vi "Manual.vi"(7 "vi reference":refnum<vi>, 8 "error in (no error)":errorcluster, 9 "IOList_280":T3, 11 "Manual":T6(tab)) -> (0 "error out":errorcluster, 3 "Out reference":refnum<vi>)   [LabVIEW 2015]
uses:
  Control Button/Exit.ctl
  Control Button/Scanner config.ctl
  Galobal variable_TI.vi
  <vilib>/Instr/_visa.llb/VISA Configure Serial Port (Instr).vi
panel:
  in  "Sensor Setting Data":T1 {"IL Sensor_Max (AI12)" format="%0.02f"; "IL Sensor_Max (AI11)" format="%0.02f"; "IL Sensor_Max (AI10)" format="%0.02f"; "IL Sensor_Max (AI9)" format="%0.02f"; "IL Sensor1_Max AI1" format="%0.02f"; "IL Sensor1_Max AI0" format="%0.02f"; "IL Sensor_Min (AI12" format="%0.02f"; "IL Sensor_Min (AI11)" format="%0.02f"; "IL Sensor_Min(AI10)" format="%0.02f"; "IL Sensor_Min  (AI9)" format="%0.02f"; "IL Sensor1_ Min AI1" format="%0.02f"; "IL Sensor1_Min AI0" format="%0.02f"}
  out "Sensor Data":T2 {"IL Sensor  (AI12" format="%0.02f"; "IL Sensor (AI11)" format="%0.02f"; "IL Sensor  (AI10)" format="%0.02f"; "IL Sensor (AI9)" format="%0.02f"; "IL Sensor1_AI1" format="%0.02f"; "IL Sensor1_AI0" format="%0.02f"}
  out "Array":string[](array[string])
  out "Byte Lenth":i32
  out "error out 2":errorcluster
  out "Manual DO":bool[](array[boolean])
  in  "Stop":T4
  out "NewVal":T5
  in  "Digital Output":T7
  out "LVDT":string
  out "Digital Input":T8
  in  "Home Calling M1":bool
  in  "Stop M1":bool
  in  "SERVO ON CMD M1":bool
  in  "Speed (mm/s) M1":i32=10
  in  "Travel (mm)M1":i32=5
  out "STM1 Done Bit":bool
  out "Error Message":string
  out "Cluster":T9
  out "Error Status":bool
  in  "Scanner config":T10
  out "Read data":string
  out "Boolean":bool
  # "Instruction for Servo motor Operate\n(1)  Switch  ON -OFF  of Fixture Slide servo Brake ON Cmd (P0.19)  \n      from Digital Output tab.\n(2) Switch  ON -OFF  of Fixture Slide Servo Direction Command (P0.20)\n      from Digital Output tab."
  # "Fixture Slide servo"
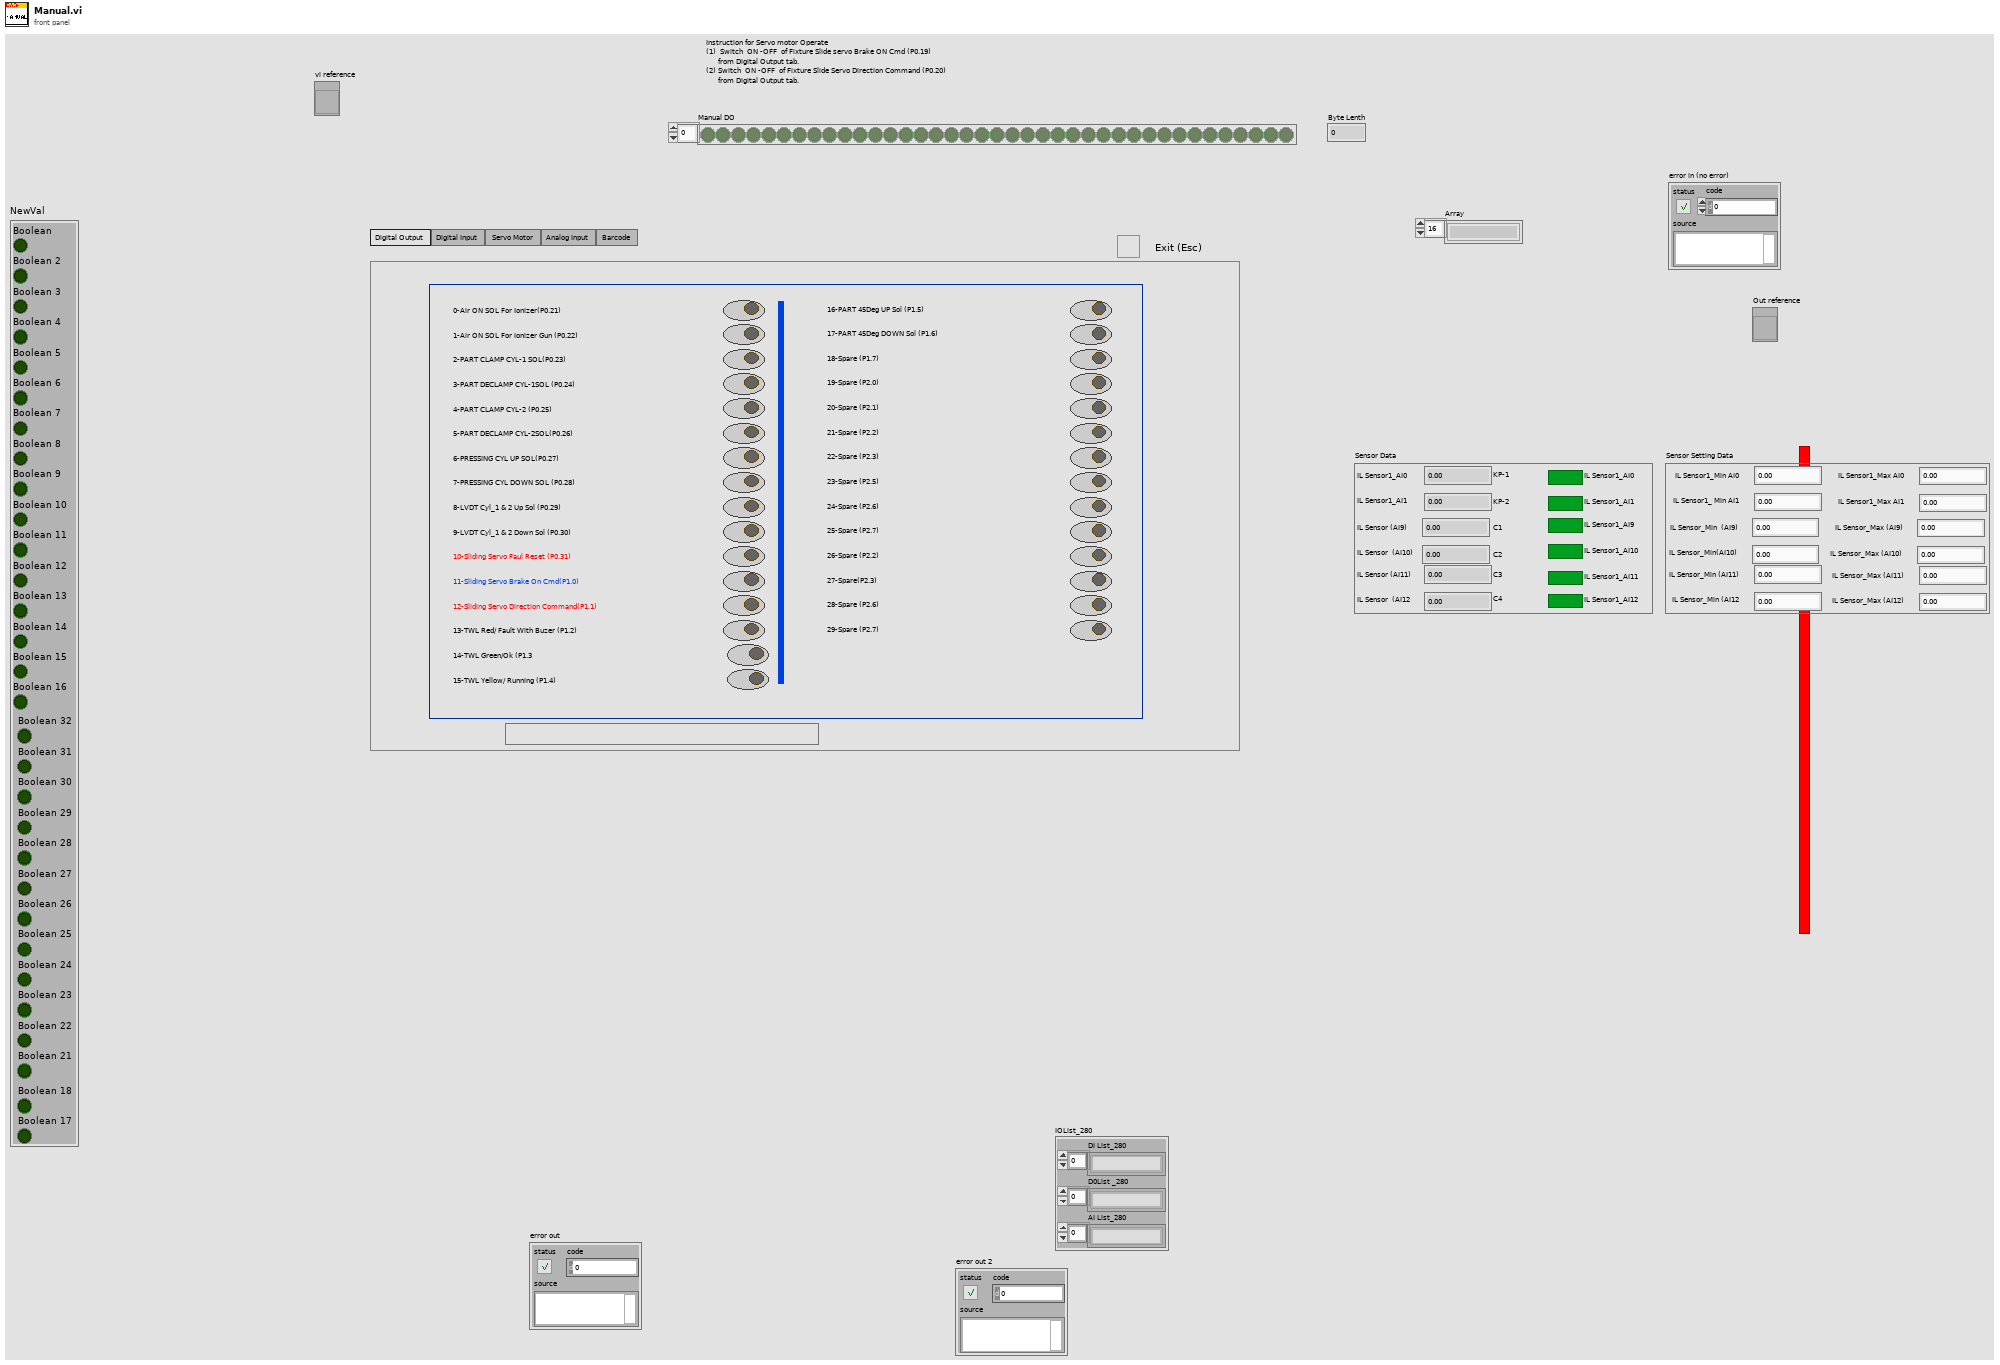
[diagram p1: front panel]
types:
  T1 = cluster{"IL Sensor1_Max AI0":dbl, "IL Sensor1_Min AI0":dbl, "IL Sensor1_Max AI1":dbl, "IL Sensor1_ Min AI1":dbl, "IL Sensor_Max (AI9)":dbl, "IL Sensor_Min  (AI9)":dbl, "IL Sensor_Max (AI10)":dbl, "IL Sensor_Min(AI10)":dbl, "IL Sensor_Max (AI11)":dbl, "IL Sensor_Min (AI11)":dbl, "IL Sensor_Max (AI12)":dbl, "IL Sensor_Min (AI12":dbl}
  T2 = cluster{"IL Sensor1_AI0":dbl, "IL Sensor1_AI1":dbl, "IL Sensor (AI9)":dbl, "IL Sensor  (AI10)":dbl, "IL Sensor (AI11)":dbl, "IL Sensor  (AI12":dbl, "IL Sensor1_AI0":bool, "IL Sensor1_AI1":bool, "IL Sensor1_AI9":bool, "IL Sensor1_AI10":bool, "IL Sensor1_AI11":bool, "IL Sensor1_AI12":bool}
  T3 = cluster{"DI List_280":string[], "D0List _280":string[], "AI List_280":string[]}
  T4 = typedef "Exit.ctl" = bool
  T5 = cluster{"Boolean":bool, "Boolean 2":bool, "Boolean 3":bool, "Boolean 4":bool, "Boolean 5":bool, "Boolean 6":bool, "Boolean 7":bool, "Boolean 8":bool, "Boolean 9":bool, "Boolean 10":bool, "Boolean 11":bool, "Boolean 12":bool, "Boolean 13":bool, "Boolean 14":bool, "Boolean 15":bool, "Boolean 16":bool, "Boolean 17":bool, "Boolean 18":bool, "Boolean 21":bool, "Boolean 22":bool, "Boolean 23":bool, "Boolean 24":bool, "Boolean 25":bool, "Boolean 26":bool, "Boolean 27":bool, "Boolean 28":bool, "Boolean 29":bool, "Boolean 30":bool, "Boolean 31":bool, "Boolean 32":bool}
  T6 = enum32{"Digital Output", "Digital Input", "Servo Motor ", "Analog Input", "Barcode "}
  T7 = cluster{"DO.00":bool, "DO.01":bool, "DO.02":bool, "DO.03":bool, "DO.04":bool, "DO.05":bool, "DO.06":bool, "DO.06":bool, "DO.07":bool, "DO.08":bool, "DO.09":bool, "DO.10":bool, "DO.11":bool, "DO.12":bool, "DO.13":bool, "DO.14":bool, "DO.07 2":bool, "DO.08 2":bool, "DO.09 2":bool, "DO.10 2":bool, "DO.11 2":bool, "DO.12 2":bool, "DO.13 2":bool, "DO.14 2":bool, "DO.00 2":bool, "DO.01 2":bool, "DO.02 2":bool, "DO.03 2":bool, "DO.06 2":bool, "DO.06 3":bool}
  T8 = cluster{"Digital Input":bool, "Digital Input 2":bool, "Digital Input 3":bool, "Digital Input 4":bool, "Digital Input 5":bool, "Digital Input 6":bool, "Digital Input 7":bool, "Digital Input 8":bool, "Digital Input 9":bool, "Digital Input 10":bool, "Digital Input 11":bool, "Digital Input 12":bool, "Digital Input 13":bool, "Digital Input 14":bool, "Digital Input 15":bool, "Digital Input 16":bool, "Digital Input 17":bool, "Digital Input 18":bool, "Digital Input 19":bool, "Digital Input 20":bool, "Digital Input 21":bool, "Digital Input 22":bool, "Digital Input 23":bool, "Digital Input 24":bool, "Digital Input 25":bool, "Digital Input 26":bool, "Digital Input 27":bool, "Digital Input 28":bool, "Digital Input 29":bool, "Digital Input 30":bool, "Digital Input 31":bool, "Digital Input 32":bool, "Digital Input 33":bool, "Digital Input 34":bool, "Digital Input 35":bool, "Digital Input 36":bool, "Digital Input 37":bool, "Digital Input 38":bool, "Digital Input 39":bool, "Digital Input 40":bool, "Digital Input 41":bool, "Digital Input 42":bool, "Digital Input 43":bool, "Digital Input 44":bool}
  T9 = cluster{"Load Cell (AI0)":dbl, "LVDT (AI1)":dbl, "LVDT (AI2)":dbl}
  T10 = typedef "Scanner config.ctl" = bool
  T11 = cluster{" Fixture Brack on":refnum<vi>, " Fixture Direction":refnum<vi>, "Servo Cmd":refnum<vi>, "Servo Home":refnum<vi>}
  T12 = cluster{"VISA resource name":refnum<visa-resource-name>, "baud rate ":u32}
  T13 = cluster{"Emergency_1":bool, "Reset_2":bool, "Home _3":bool, "Air Pressure_4":bool, "Safety Sensor_5":bool, "Safety Sensor_6":bool, "Slide Servo Home RS 26":bool, "LVDT UP RS":bool, "Servo Fault 27":bool, "Pressing UP RS 31":bool, "40 Deg. Down Fixture Rs":bool}
  T14 = cluster{"IL Sensor1_AI0":dbl, "IL Sensor1_AI1":dbl, "IL Sensor (AI6)":dbl, "IL Sensor  (AI7)":dbl, "IL Sensor (AI8)":dbl, "IL Sensor  (AI9)":dbl, "IL Sensor1_AI0":bool, "IL Sensor1_AI1":bool, "IL Sensor1_AI9":bool, "IL Sensor1_AI10":bool, "IL Sensor1_AI11":bool, "IL Sensor1_AI12":bool}
  T15 = cluster{"Digital input[0]":bool, "Digital input[1]":bool, "Digital input[2]":bool, "Digital input[3]":bool, "Digital input[4]":bool, "Digital input[5]":bool, "Digital input[6]":bool, "Digital input[7]":bool, "Digital input[8]":bool, "Digital input[9]":bool, "Digital input[10]":bool, "Digital input[11]":bool, "Digital input[12]":bool, "Digital input[13]":bool, "Digital input[14]":bool, "Digital input[15]":bool, "Digital input[16]":bool, "Digital input[17]":bool, "Digital input[18]":bool, "Digital input[19]":bool, "Digital input[20]":bool, "Digital input[21]":bool, "Digital input[22]":bool, "Digital input[23]":bool, "Digital input[24]":bool, "Digital input[25]":bool, "Digital input[26]":bool, "Digital input[27]":bool, "Digital input[28]":bool, "Digital input[29]":bool, "Digital input[30]":bool, "Digital input[31]":bool, "Digital input[32]":bool, "Digital input[33]":bool, "Digital input[34]":bool, "Digital input[35]":bool, "Digital input[36]":bool, "Digital input[37]":bool, "Digital input[38]":bool, "Digital input[39]":bool, "Digital input[40]":bool, "Digital input[41]":bool, "Digital input[42]":bool, "Digital input[43]":bool}
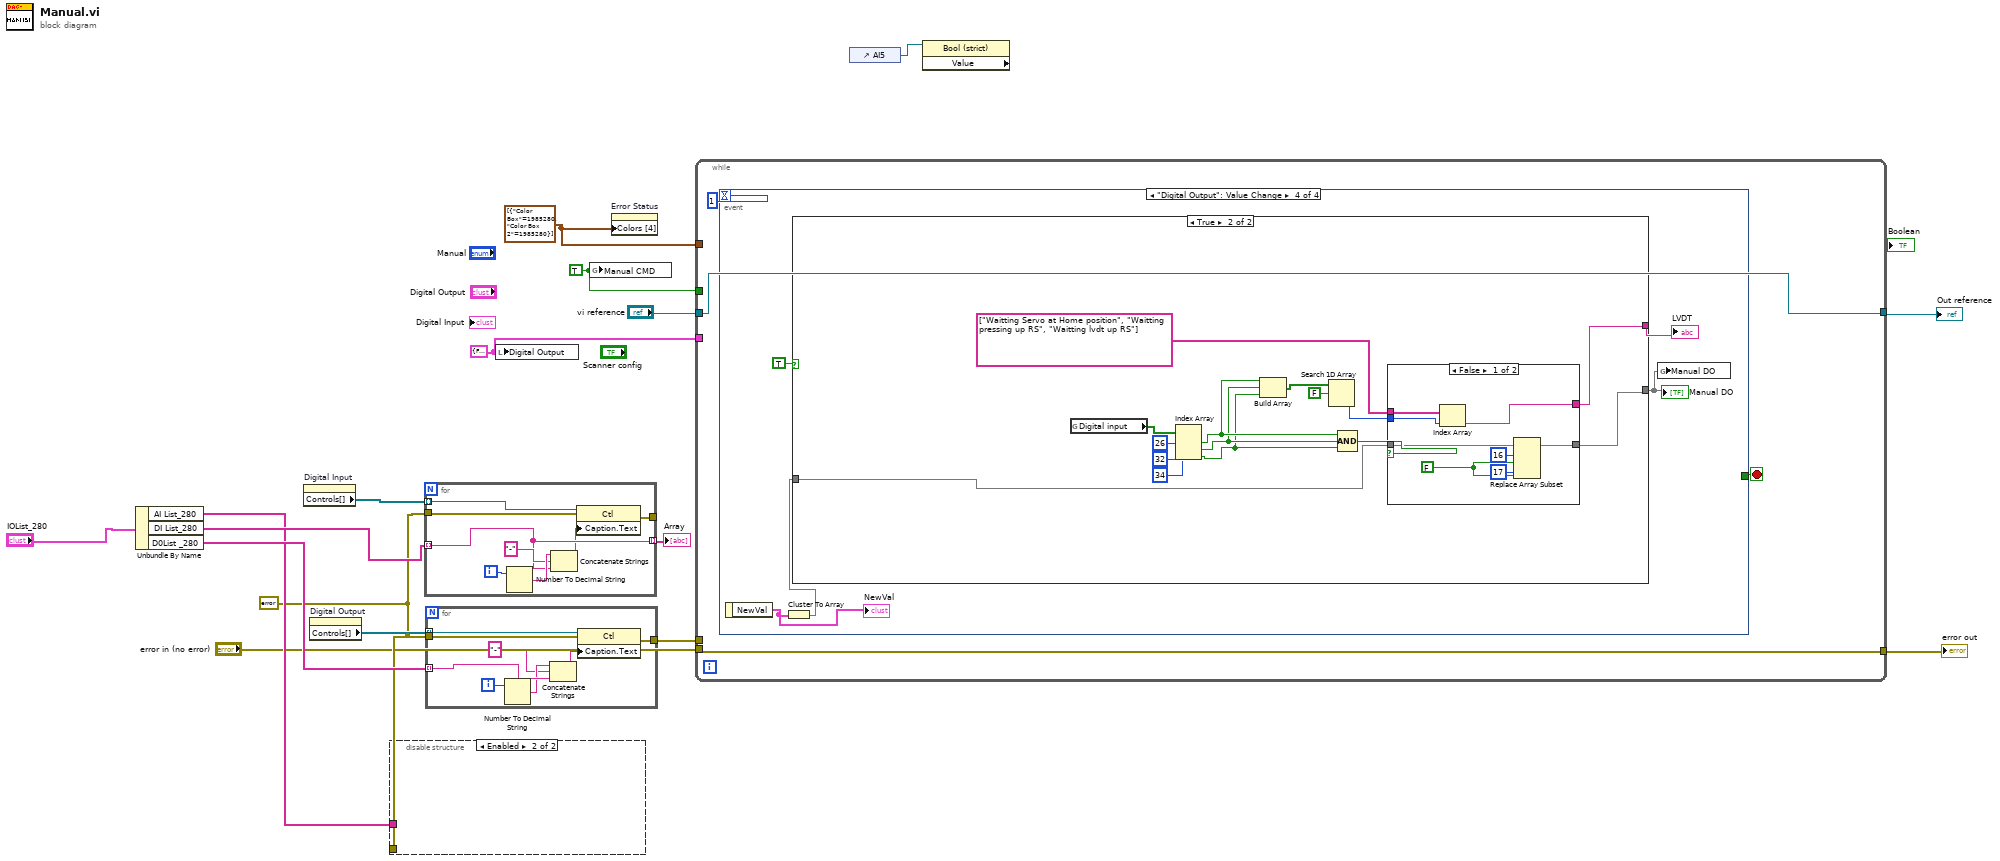
[diagram p0: block diagram]
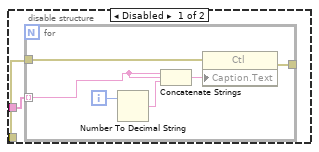
[diagram p2: hidden frame]
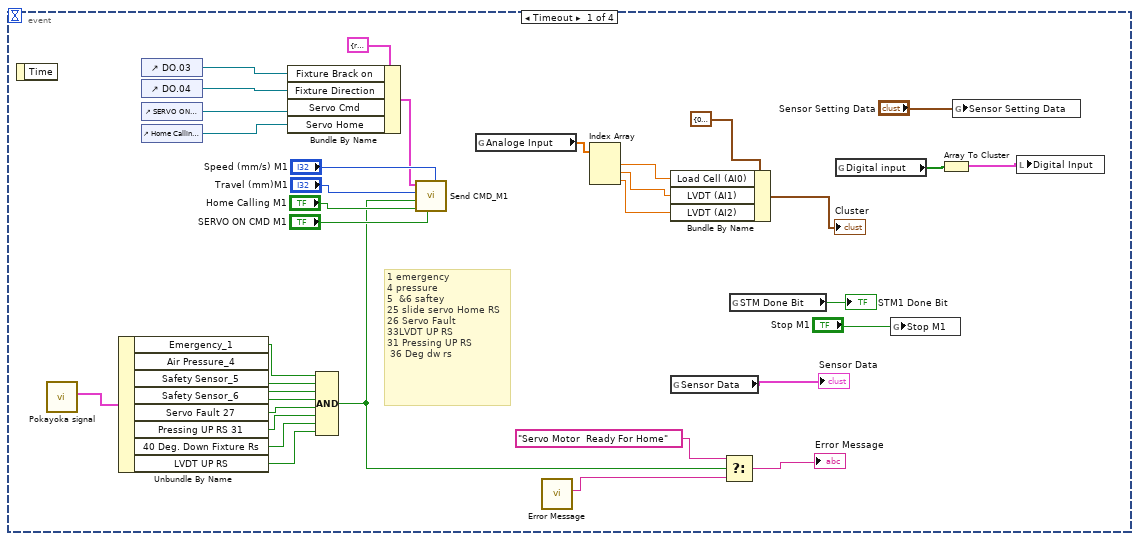
[diagram p3: hidden frame]
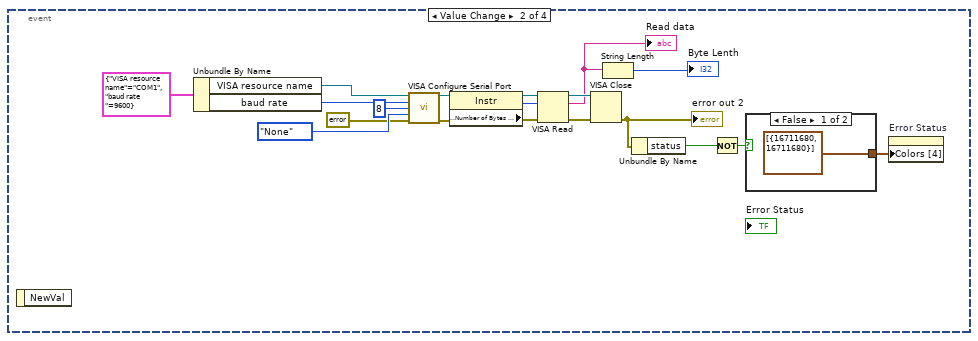
[diagram p4: hidden frame]
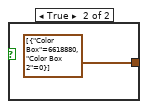
[diagram p5: hidden frame]
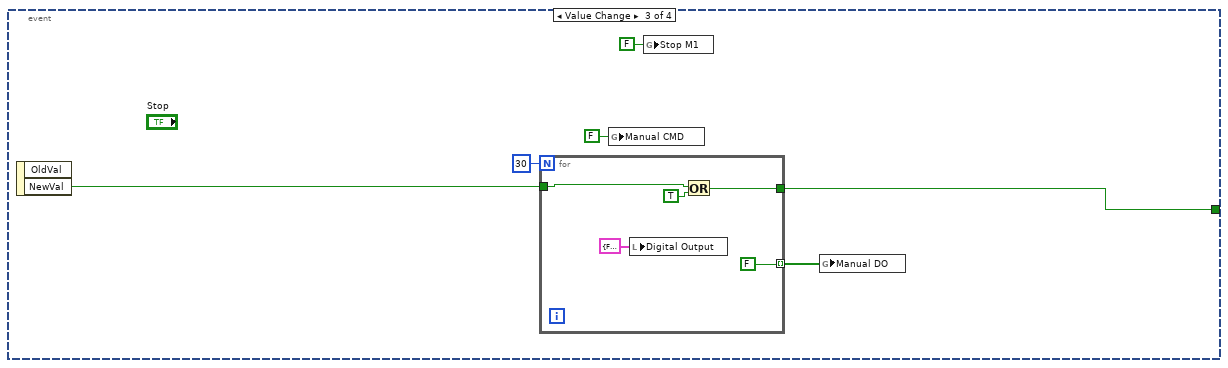
[diagram p6: hidden frame]
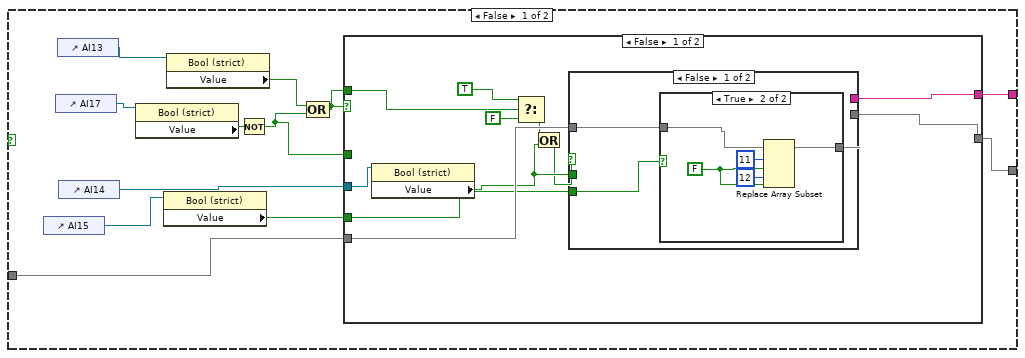
[diagram p7: hidden frame]
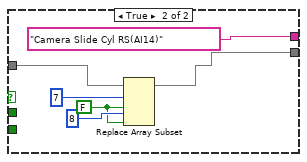
[diagram p9: hidden frame]
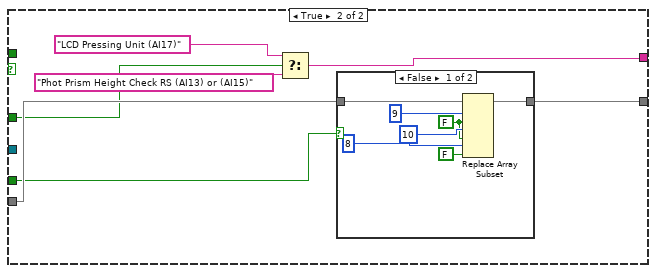
[diagram p10: hidden frame]
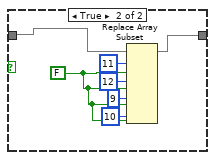
[diagram p11: hidden frame]
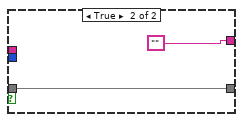
[diagram p12: hidden frame]
diagram:
  w2 = T7 {"DO.00"=FALSE, "DO.01"=FALSE, "DO.02"=FALSE, "DO.03"=FALSE, "DO.04"=FALSE, "DO.05"=FALSE, "DO.06"=FALSE, "DO.06"=FALSE, "DO.07"=FALSE, "DO.08"=FALSE, "DO.09"=FALSE, "DO.10"=FALSE, "DO.11"=FALSE, "DO.12"=FALSE, "DO.13"=FALSE, "DO.14"=FALSE, "DO.07 2"=FALSE, "DO.08 2"=FALSE, "DO.09 2"=FALSE, "DO.10 2"=FALSE, "DO.11 2"=FALSE, "DO.12 2"=FALSE, "DO.13 2"=FALSE, "DO.14 2"=FALSE, "DO.00 2"=FALSE, "DO.01 2"=FALSE, "DO.02 2"=FALSE, "DO.03 2"=FALSE, "DO.06 2"=FALSE, "DO.06 3"=FALSE} ("Digital Output")
  w5 = errorcluster {"status"=FALSE, "code"=0, "source"=""} ("error in (no error)")
  w8 = cluster{"Color Box":u32, "Color Box 2":u32}[] [{"Color Box"=1985280, "Color Box 2"=1985280}] ("Colors [4]")
  w13 = TRUE ("Manual CMD")
  n1 = Unbundle By Name("IOList_280") -> ("AI List_280"=w9:string[], "DI List_280"=w10:string[], "D0List _280"=w12:string[])
  n2 = property on="Digital Input" class="Clust (strict)"() -> ("Controls[]"=w11:refnum<vi>[])  [unwired: 2 in, 2 out]
  n3 = property on="Digital Output" class="Clust (strict)"() -> ("Controls[]"=w16:refnum<vi>[])  [unwired: 2 in, 2 out]
  n4 = disable-structure shown="Enabled" {
    disable-tunnel: w9 -> [w19 _]
    disable-tunnel: w5 -> [w18 _]
    frame Disabled {
      n5 = for {
        tunnel: [w23] -> _
        tunnel: w18 -> [w21]
        tunnel: w19 -> [w20] mode=indexing
        i -> [w24]
        n6 = Number To Decimal String(number=w24) -> (decimal integer string=w22:string)  [unwired: 1 in]
        n7 = Concatenate Strings(w20, w22) -> ()  [unwired: 1 out]
        n8 = property class="Ctl"(error in=w21, "Caption.Text"=w20) -> (error out=w23:errorcluster)  [unwired: 1 in, 1 out]
      }
    }
    frame Enabled {
    }
  }
  n9 = for {
    tunnel: w11 -> [w32] mode=indexing
    tunnel: [w30] -> _
    tunnel: w5 -> [w29]
    tunnel: w10 -> [w26] mode=indexing
    tunnel: [w26] -> w6 mode=indexing
    i -> [w31]
    n10 = Number To Decimal String(number=w31) -> (decimal integer string=w28:string)  [unwired: 1 in]
    n11 = Concatenate Strings(w28, "-" ("string"), w26) -> (w25:string)
    n12 = property class="Ctl"(reference=w32, error in=w29, "Caption.Text"=w25) -> (error out=w30:errorcluster)  [unwired: 1 out]
  }
  "Array" <- w6
  n13 = for {
    tunnel: w16 -> [w40] mode=indexing
    tunnel: [w38] -> w17
    tunnel: w5 -> [w37]
    tunnel: w12 -> [w36] mode=indexing
    i -> [w39]
    n14 = Number To Decimal String(number=w39) -> (decimal integer string=w35:string)  [unwired: 1 in]
    n15 = Concatenate Strings(w35, "-" ("string"), w36) -> (w33:string)
    n16 = property class="Ctl"(reference=w40, error in=w37, "Caption.Text"=w33) -> (error out=w38:errorcluster)  [unwired: 1 out]
  }
  n17 = local write "Digital Output"(w2) -> ()
  n18 = global write "Galobal variable_TI.vi" "Manual CMD"(w13) -> ()
  n19 = property on="Error Status" class="Bool (strict)"("Colors [4]"=w8) -> ()  [unwired: 2 in, 2 out]
  n20 = while {
    tunnel: w17 -> [_]
    tunnel: [w42] -> w15
    tunnel: "vi reference" -> [w43]
    tunnel: [w43] -> w14
    tunnel: w13 -> [_]
    tunnel: w8 -> [_]
    tunnel: "error in (no error)" -> [w42]
    tunnel: w2 -> [_]
    stop <- w41 stop-if-true
    n21 = event shown="[3] \"Digital Output\": Value Change" {
      selector: _ -> [_ _ _ _]
      dyn-events: _ -> [_ _ _ _]
      timeout: 1 -> [_ _ _ _]
      tunnel: [_ _ w101 _] -> w41
      event Timeout {
        # "1 emergency\n4 pressure\n5  &6 saftey\n25 slide servo Home RS\n26 Servo Fault\n33LVDT UP RS\n31 Pressing UP RS \n 36 Deg dw rs"
        n22 = event-data() -> ()  [unwired: 1 in, 1 out]
        n23 = call "Pokayoka signal.vi"() -> ("output cluster"=w60:T13)  [unwired: 10 in, 1 out]
        n24 = Unbundle By Name(w60) -> ("Emergency_1"=w54:bool, "Air Pressure_4"=w59:bool, "Safety Sensor_5"=w58:bool, "Safety Sensor_6"=w57:bool, "Servo Fault 27"=w56:bool, "Pressing UP RS 31"=w53:bool, "40 Deg. Down Fixture Rs"=w52:bool, "LVDT UP RS"=w51:bool)
        n25 = control-ref of="DO.03"() -> (w72:refnum<vi>)
        n26 = control-ref of="DO.04"() -> (w71:refnum<vi>)
        n27 = control-ref of="SERVO ON CMD M1"() -> (w69:refnum<vi>)
        n28 = control-ref of="Home Calling M1"() -> (w70:refnum<vi>)
        n29 = Bundle By Name(cluster=T11 {" Fixture Brack on"=refnum, " Fixture Direction"=refnum, "Servo Cmd"=refnum, "Servo Home"=refnum} ("Slide Servo"), "Fixture Brack on"=w72, "Fixture Direction"=w71, "Servo Cmd"=w69, "Servo Home"=w70) -> (w68:T11)
        n30 = Compound Arithmetic op=AND(w54, w59, w58, w57, w56, w53, w52, w51) -> (w55:bool)
        n31 = call "Send CMD_M1.vi"("Speed (mm/s) M1"="Speed (mm/s) M1", "SERVO ON CMD M1"="SERVO ON CMD M1", "Home Calling M1"="Home Calling M1", "Pokayoka"=w55, "Travel (mm)M1"="Travel (mm)M1", "Slide Servo"=w68) -> ()  [unwired: 6 in]
        n32 = global read "Galobal variable_TI.vi" "Analoge Input"() -> (w50:dbl[])
        n33 = call "Error Message.vi"() -> ("Error"=w64:string)  [unwired: 10 in, 1 out]
        n34 = Index Array(array=w50) -> (element #1=w48:dbl, element #2=w47:dbl, element #3=w46:dbl)  [unwired: 3 in]
        n35 = Bundle By Name(cluster=T9 {"Load Cell (AI0)"=0.0, "LVDT (AI1)"=0.0, "LVDT (AI2)"=0.0} ("Cluster 2"), "Load Cell (AI0)"=w48, "LVDT (AI1)"=w47, "LVDT (AI2)"=w46) -> (→"Cluster":T9)
        n36 = global read "Galobal variable_TI.vi" "Sensor Data"() -> (→"Sensor Data":T14)
        n37 = Select(t="Servo Motor  Ready For Home", s=w55, f=w64) -> (s? t:f=→"Error Message":string)
        n38 = global read "Galobal variable_TI.vi" "STM Done Bit"() -> (→"STM1 Done Bit":bool)
        n39 = global read "Galobal variable_TI.vi" "Digital input"() -> (w67:bool[])
        n40 = global write "Galobal variable_TI.vi" "Stop M1"("Stop M1") -> ()
        n41 = Array To Cluster(array=w67) -> (cluster=w79:T15)
        n42 = global write "Galobal variable_TI.vi" "Sensor Setting Data"("Sensor Setting Data") -> ()
        n43 = local write "Digital Input"(w79) -> ()
      }
      event Value Change {
        n44 = event-data() -> ()  [unwired: 1 in, 1 out]
        n45 = Unbundle By Name(T12 {"VISA resource name"="COM1", "baud rate "=9600} ("Cluster")) -> ("VISA resource name"=w98:refnum<visa-resource-name>, "baud rate"=w97:u32)
        n46 = call-poly "VISA Configure Serial Port"("VISA resource name"=w98, "baud rate (9600)"=w97, "data bits (8)"=u16 8, "parity (0:none)"=enum16{"None", "Odd", "Even", "Mark", "Space"}."None", "error in (no error)"=errorcluster {"status"=FALSE, "code"=0, "source"=""} ("error in (no error) 2")) -> ("VISA resource name out"=w96:refnum<visa-resource-name>, "error out"=w94:errorcluster)  [unwired: 9 in]
        n47 = property class="Instr"(reference=w96, error in=w94) -> (reference out=w95:refnum<visa-resource-name>, error out=w93:errorcluster, "Serial Settings:Number of Bytes at Serial Port"=w92:u32)
        n48 = VISA Read(VISA resource name=w95, byte count=w92, error in (no error)=w93) -> (VISA resource name out=w90:refnum<visa-resource-name>, read buffer=w88:string, error out=w89:errorcluster)  [unwired: 1 out]
        "Read data" <- w88
        n49 = VISA Close(VISA resource name=w90, error in (no error)=w89) -> (error out=w86:errorcluster)
        "error out 2" <- w86
        n50 = String Length(string=w88) -> (length=→"Byte Lenth":i32)
        n51 = Unbundle By Name(w86) -> ("status"=w85:bool)
        n52 = Not(x=w85) -> (.not. x?=w83:bool)
        n53 = case shown="False" w83 {
          tunnel: [cluster{"Color Box":u32, "Color Box 2":u32}[] [{"Color Box"=16711680, "Color Box 2"=16711680}] ("Colors [4]") cluster{"Color Box":u32, "Color Box 2":u32}[] [{"Color Box"=6618880, "Color Box 2"=0}] ("Colors [4]")] -> w84
          frame False {
          }
          frame True {
          }
        }
        n54 = property on="Error Status" class="Bool (strict)"("Colors [4]"=w84) -> ()  [unwired: 2 in, 2 out]
      }
      event Value Change {
        n55 = event-data() -> ("NewVal"=w102:T4)  [unwired: 1 in, 1 out]
        n56 = for {
          N: 30 -> [_]
          tunnel: [FALSE] -> w104 mode=indexing
          tunnel: w102 -> [w109]
          tunnel: [w108] -> w101
          n57 = local write "Digital Output"(T7 {"DO.00"=FALSE, "DO.01"=FALSE, "DO.02"=FALSE, "DO.03"=FALSE, "DO.04"=FALSE, "DO.05"=FALSE, "DO.06"=FALSE, "DO.06"=FALSE, "DO.07"=FALSE, "DO.08"=FALSE, "DO.09"=FALSE, "DO.10"=FALSE, "DO.11"=FALSE, "DO.12"=FALSE, "DO.13"=FALSE, "DO.14"=FALSE, "DO.07 2"=FALSE, "DO.08 2"=FALSE, "DO.09 2"=FALSE, "DO.10 2"=FALSE, "DO.11 2"=FALSE, "DO.12 2"=FALSE, "DO.13 2"=FALSE, "DO.14 2"=FALSE, "DO.00 2"=FALSE, "DO.01 2"=FALSE, "DO.02 2"=FALSE, "DO.03 2"=FALSE, "DO.06 2"=FALSE, "DO.06 3"=FALSE} ("Digital Output")) -> ()
          n58 = Or(x=w109, y=TRUE) -> (x .or. y?=w108:T4)
        }
        n59 = global write "Galobal variable_TI.vi" "Manual CMD"(FALSE ("Manual CMD")) -> ()
        n60 = global write "Galobal variable_TI.vi" "Stop M1"(FALSE ("Stop M1")) -> ()
        n61 = global write "Galobal variable_TI.vi" "Manual DO"(w104) -> ()
      }
      event "Digital Output": Value Change {
        n62 = event-data() -> ("NewVal"=w112:T7)  [unwired: 1 in]
        "NewVal" <- w112
        n63 = Cluster To Array(cluster=w112) -> (array=w113:bool[])
        n64 = case shown="True" TRUE ("By Pass") {
          tunnel: [w127 w184] -> w116
          tunnel: [w125 w183] -> w115
          tunnel: w113 -> [w118 w186]
          frame False {
            n65 = control-ref of="AI15"() -> (w119:refnum<vi>)
            n66 = control-ref of="AI17"() -> (w122:refnum<vi>)
            n67 = control-ref of="AI13"() -> (w126:refnum<vi>)
            n68 = control-ref of="AI14"() -> (w128:refnum<vi>)
            n69 = property class="Bool (strict)"(reference=w122) -> ("Value"=w123:bool)  [unwired: 1 in, 2 out]
            n70 = property class="Bool (strict)"(reference=w119) -> ("Value"=w117:bool)  [unwired: 1 in, 2 out]
            n71 = property class="Bool (strict)"(reference=w126) -> ("Value"=w124:bool)  [unwired: 1 in, 2 out]
            n72 = Not(x=w123) -> (.not. x?=w121:bool)
            n73 = Compound Arithmetic op=OR(w124, w121) -> (w120:bool)
            n74 = case shown="False" w120 {
              tunnel: w118 -> [w139 w161]
              tunnel: w128 -> [w138 _]
              tunnel: [w129 w160] -> w127
              tunnel: [w137 w156] -> w125
              tunnel: w121 -> [_ w159]
              tunnel: w120 -> [w136 _]
              tunnel: w117 -> [w130 w155]
              frame False {
                n75 = property class="Bool (strict)"(reference=w138) -> ("Value"=w132:bool)  [unwired: 1 in, 2 out]
                n76 = Select(t=TRUE, s=w136, f=FALSE) -> (s? t:f=w133:bool)
                n77 = Or(x=w133, y=w132) -> (x .or. y?=w131:bool)
                n78 = case shown="False" w131 {
                  tunnel: w139 -> [w141 w152]
                  tunnel: [w140 w151] -> w129
                  tunnel: w132 -> [_ _]
                  tunnel: [_ "Camera Slide Cyl RS(AI14)"] -> w137
                  tunnel: w130 -> [w142 _]
                  frame False {
                    n79 = case shown="True" w142 {
                      tunnel: w141 -> [w143 w146]
                      tunnel: [w143 w145] -> w140
                      frame False {
                      }
                      frame True {
                        w144 = FALSE ("new element/subarray")
                        n80 = Replace Array Subset(array=w146, new element #1=w144, index #1=11 ("index"), new element #2=w144, index #2=12 ("index")) -> (w145:bool[])
                      }
                    }
                  }
                  frame True {
                    w149 = FALSE ("new element/subarray")
                    n81 = Replace Array Subset(array=w152, new element #1=w149, index #1=7 ("index"), new element #2=w149, index #2=8 ("index")) -> (w151:bool[])
                  }
                }
              }
              frame True {
                n82 = Select(t="LCD Pressing Unit (AI17)", s=w159, f="Phot Prism Height Check RS (AI13) or (AI15)") -> (s? t:f=w156:string)
                n83 = case shown="False" w155 {
                  tunnel: w161 -> [w165 w173]
                  tunnel: [w164 w172] -> w160
                  frame False {
                    w166 = FALSE ("new element/subarray")
                    n84 = Replace Array Subset(array=w165, new element #1=w166, index #1=9 ("index"), new element #2=w166, index #2=10 ("index"), new element #3=FALSE ("new element/subarray"), index #3=8 ("index")) -> (w164:bool[])
                  }
                  frame True {
                    w169 = FALSE ("new element/subarray")
                    n85 = Replace Array Subset(array=w173, new element #1=w169, index #1=11 ("index"), new element #2=w169, index #2=12 ("index"), new element #3=w169, index #3=9 ("index"), new element #4=w169, index #4=10 ("index")) -> (w172:bool[])
                  }
                }
              }
            }
          }
          frame True {
            n86 = global read "Galobal variable_TI.vi" "Digital input"() -> (w190:bool[])
            n87 = Index Array(array=w190, index #1=26 ("index"), index #2=32 ("index"), index #3=34 ("index")) -> (element #1=w182:bool, element #2=w181:bool, element #3=w180:bool)
            n88 = Build Array(w182, w181, w180) -> (w179:bool[])
            n89 = Search 1D Array(1D array=w179, element=FALSE) -> (index of element=w176:i32)  [unwired: 1 in]
            n90 = Compound Arithmetic op=AND(w182, w181, w180) -> (w185:bool)
            n91 = case shown="False" w185 {
              tunnel: w186 -> [w198 w200]
              tunnel: [w197 w200] -> w184
              tunnel: [w194 ""] -> w183
              tunnel: string[] ["Waitting Servo at Home position", "Waitting pressing up RS", "Waitting lvdt up RS"] -> [w196 _]
              tunnel: w176 -> [w195 _]
              frame False {
                w191 = FALSE ("new element/subarray")
                n92 = Index Array(array=w196, index=w195) -> (element=w194:string)
                n93 = Replace Array Subset(array=w198, new element #1=w191, index #1=16 ("index"), new element #2=w191, index #2=17 ("index")) -> (w197:bool[])
              }
              frame True {
              }
            }
          }
        }
        "Manual DO" <- w116
        "LVDT" <- w115
        n94 = global write "Galobal variable_TI.vi" "Manual DO"(w116) -> ()
      }
    }
  }
  "error out" <- w15
  "Out reference" <- w14
  n95 = control-ref of="AI5"() -> (w1:refnum<vi>)
  n96 = property class="Bool (strict)" props=["Value"](reference=w1) -> ()  [unwired: 1 in, 3 out]
